vi "interfaz-grafica.vi"() -> ()   [LabVIEW 2024]
uses:
  TG JD - running/TG Juan Diego/Documentos de Labview/160620 Optotune Lens Driver 4 Labview package/Hello Optotune Lens (30.06.2015)/Calibration.ctl
  <vilib>/Instr/_visa.llb/VISA Configure Serial Port (Instr).vi
  <vilib>/Utility/file.llb/Write Delimited Spreadsheet (string).vi
  <vilib>/Utility/file.llb/Read Delimited Spreadsheet (string).vi
  <vilib>/vision/NI_Vision_Development_Module.lvlib
panel:
  out "Path Video":path
  out "Path Potencia Optica D":path
  out "Path Potencia Optica I":path
  in  "stop":bool
  out "Array 2":dbl[](array[numeric])
  out "Array":dbl[](array[numeric])
  out "Path DATOS":path
  in  "stop 2":bool
  out "Path":path=path "C:/Users/willi/GITHUB/TG/OBJ 2 - RECOLECCION DE DATOS/registro-usuarios.csv"
  out "error out":errorcluster
  in  "Tab Control":enum32{"Experimento", "Configuración"}(tab)
  in  "ADQUIRIR":bool
  in  "DETENER":bool
  out "DPT  IZQ":dbl
  out "DPT  DER":dbl
  out "Potencia  Ojo Derecho":dbl[](graph)
  out "ROI (Ojo)":T1(plugin-control)
  out "Path ADQUISICION":path
  out "Usuario seleccionado":string caption="USUARIO"
  in  "Potencia inicial lente derecho":dbl(slide) scale=-3.0..3.0
  in  "Potencia inicial lente izquierdo":dbl(slide) scale=-3.0..3.0
  out "Full Image":T1(plugin-control)
  in  "VISA resource name 3":refnum<visa-resource-name>
  in  "Tab Control 2":T2(tab)
  in  "Usuario":string(combo)
  in  "registrarButtom":bool
  in  "Cluster":T3 {"Fecha de nacimiento" format="%<%x>T"}
  out "Nuevo Usuario":i32
  out "USUARIO":string
  in  "VISA resource name 4":refnum<visa-resource-name>
  out "error out 4":errorcluster
  out "error out 3":errorcluster
  in  "stop 4":bool
  in  "error in (no error) 3":errorcluster
  in  "error in (no error) 4":errorcluster
  in  "stop 3":bool
  out "VISA resource name out 2":string
  out "Command to Port":string
  out "Data":string
  out "OK":bool
  out "Calibration 2":T4 {"Max Current A" format="%#_g mA"; "Max Current B" format="%#_g mA"; "UCL A" format="%#_g mA"; "LCL A" format="%#_g mA"; "UCL B" format="%#_g mA"; "LCL B" format="%#_g mA"}
  out "VISA resource name out":string
  out "ID":u16
  in  "Calibration":T4={"Max Current A"=293.0, "Max Current B"=293.0, "UCL A"=300.0, "UCL B"=300.0, "LCL A"=0.0, "LCL B"=0.0} {"Max Current A" format="%#_g mA"; "Max Current B" format="%#_g mA"; "UCL A" format="%#_g mA"; "LCL A" format="%#_g mA"; "UCL B" format="%#_g mA"; "LCL B" format="%#_g mA"}
  # "Seleccione la Region de Interes (ROI. el ojo)"
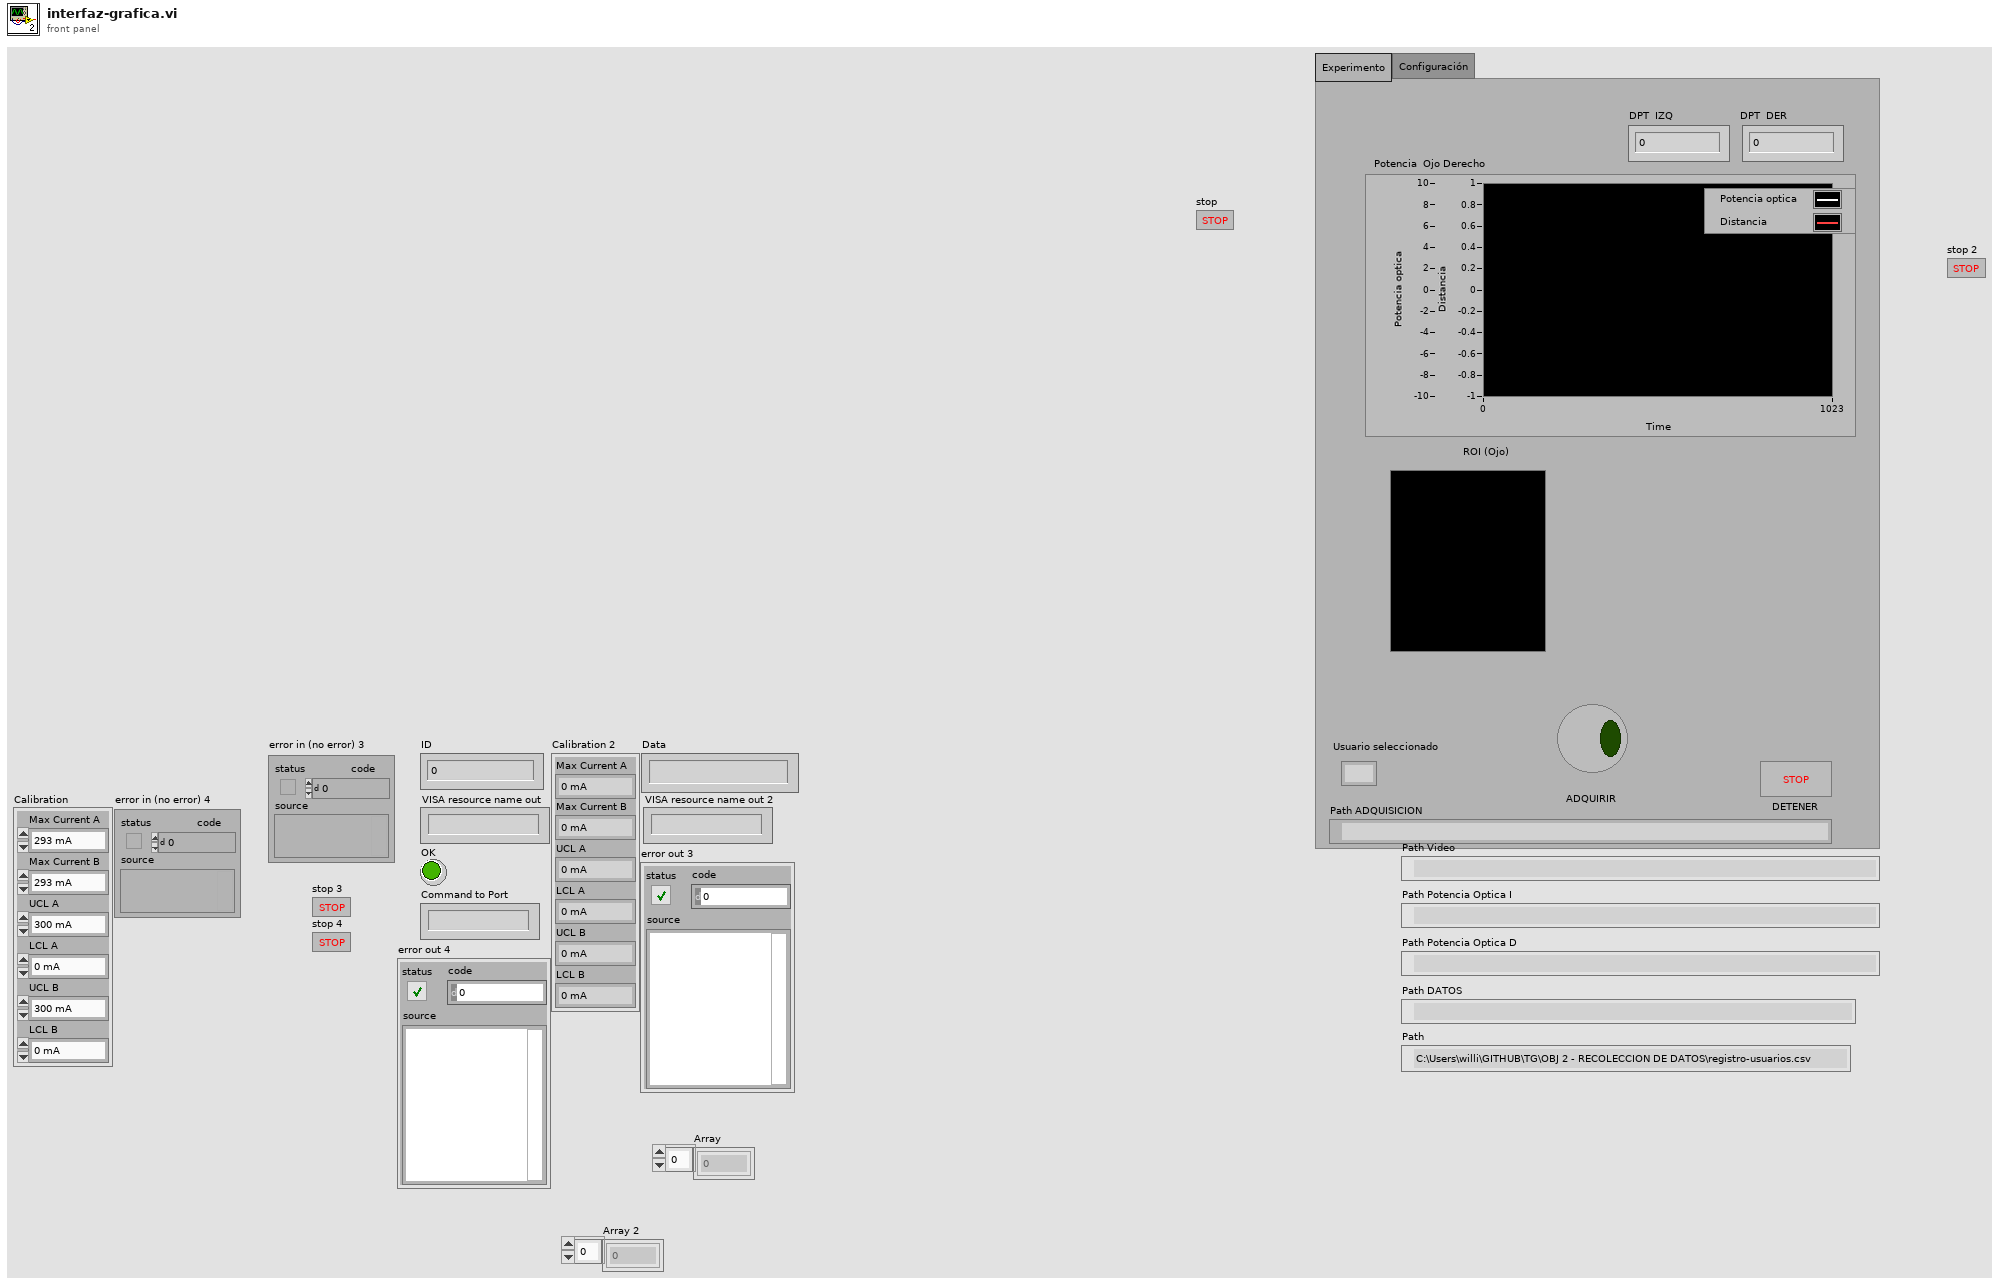
[diagram p1: front panel]
types:
  T1 = typedef "IMAQ Image.ctl" = refnum<image>
  T2 = enum32{"Seleccionar Usuario", "Registrar Nuevo Usuario"}
  T3 = cluster{"Fecha de nacimiento":timestamp, "Genero":enum16{"Mujer", "Hombre"}, "Error Refractivo":enum16{"No sabe", "Miopia", "Hipermetropia", "No tiene"}}
  T4 = typedef "Calibration.ctl" = cluster{"Max Current A":dbl, "Max Current B":dbl, "UCL A":dbl, "UCL B":dbl, "LCL A":dbl, "LCL B":dbl}
  T5 = typedef "Image Type" = u32
  T6 = cluster{"Numero \nUsuario":i32, "Fecha de nacimiento":timestamp, "Genero":enum16{"Mujer", "Hombre"}, "Error Refractivo":enum16{"No sabe", "Miopia", "Hipermetropia", "No tiene"}}
  T7 = enum16{"No sabe", "Miopia", "Hipermetropia", "No tiene"}
  T8 = cluster{"Global Rectangle":i32[], "Contours":cluster{"Contour Type":u32, "ROI Type":u32, "Points":i32[]}[]}
  T9 = typedef "IMAQ AVI2 Refnum.ctl" = refnum<k20>
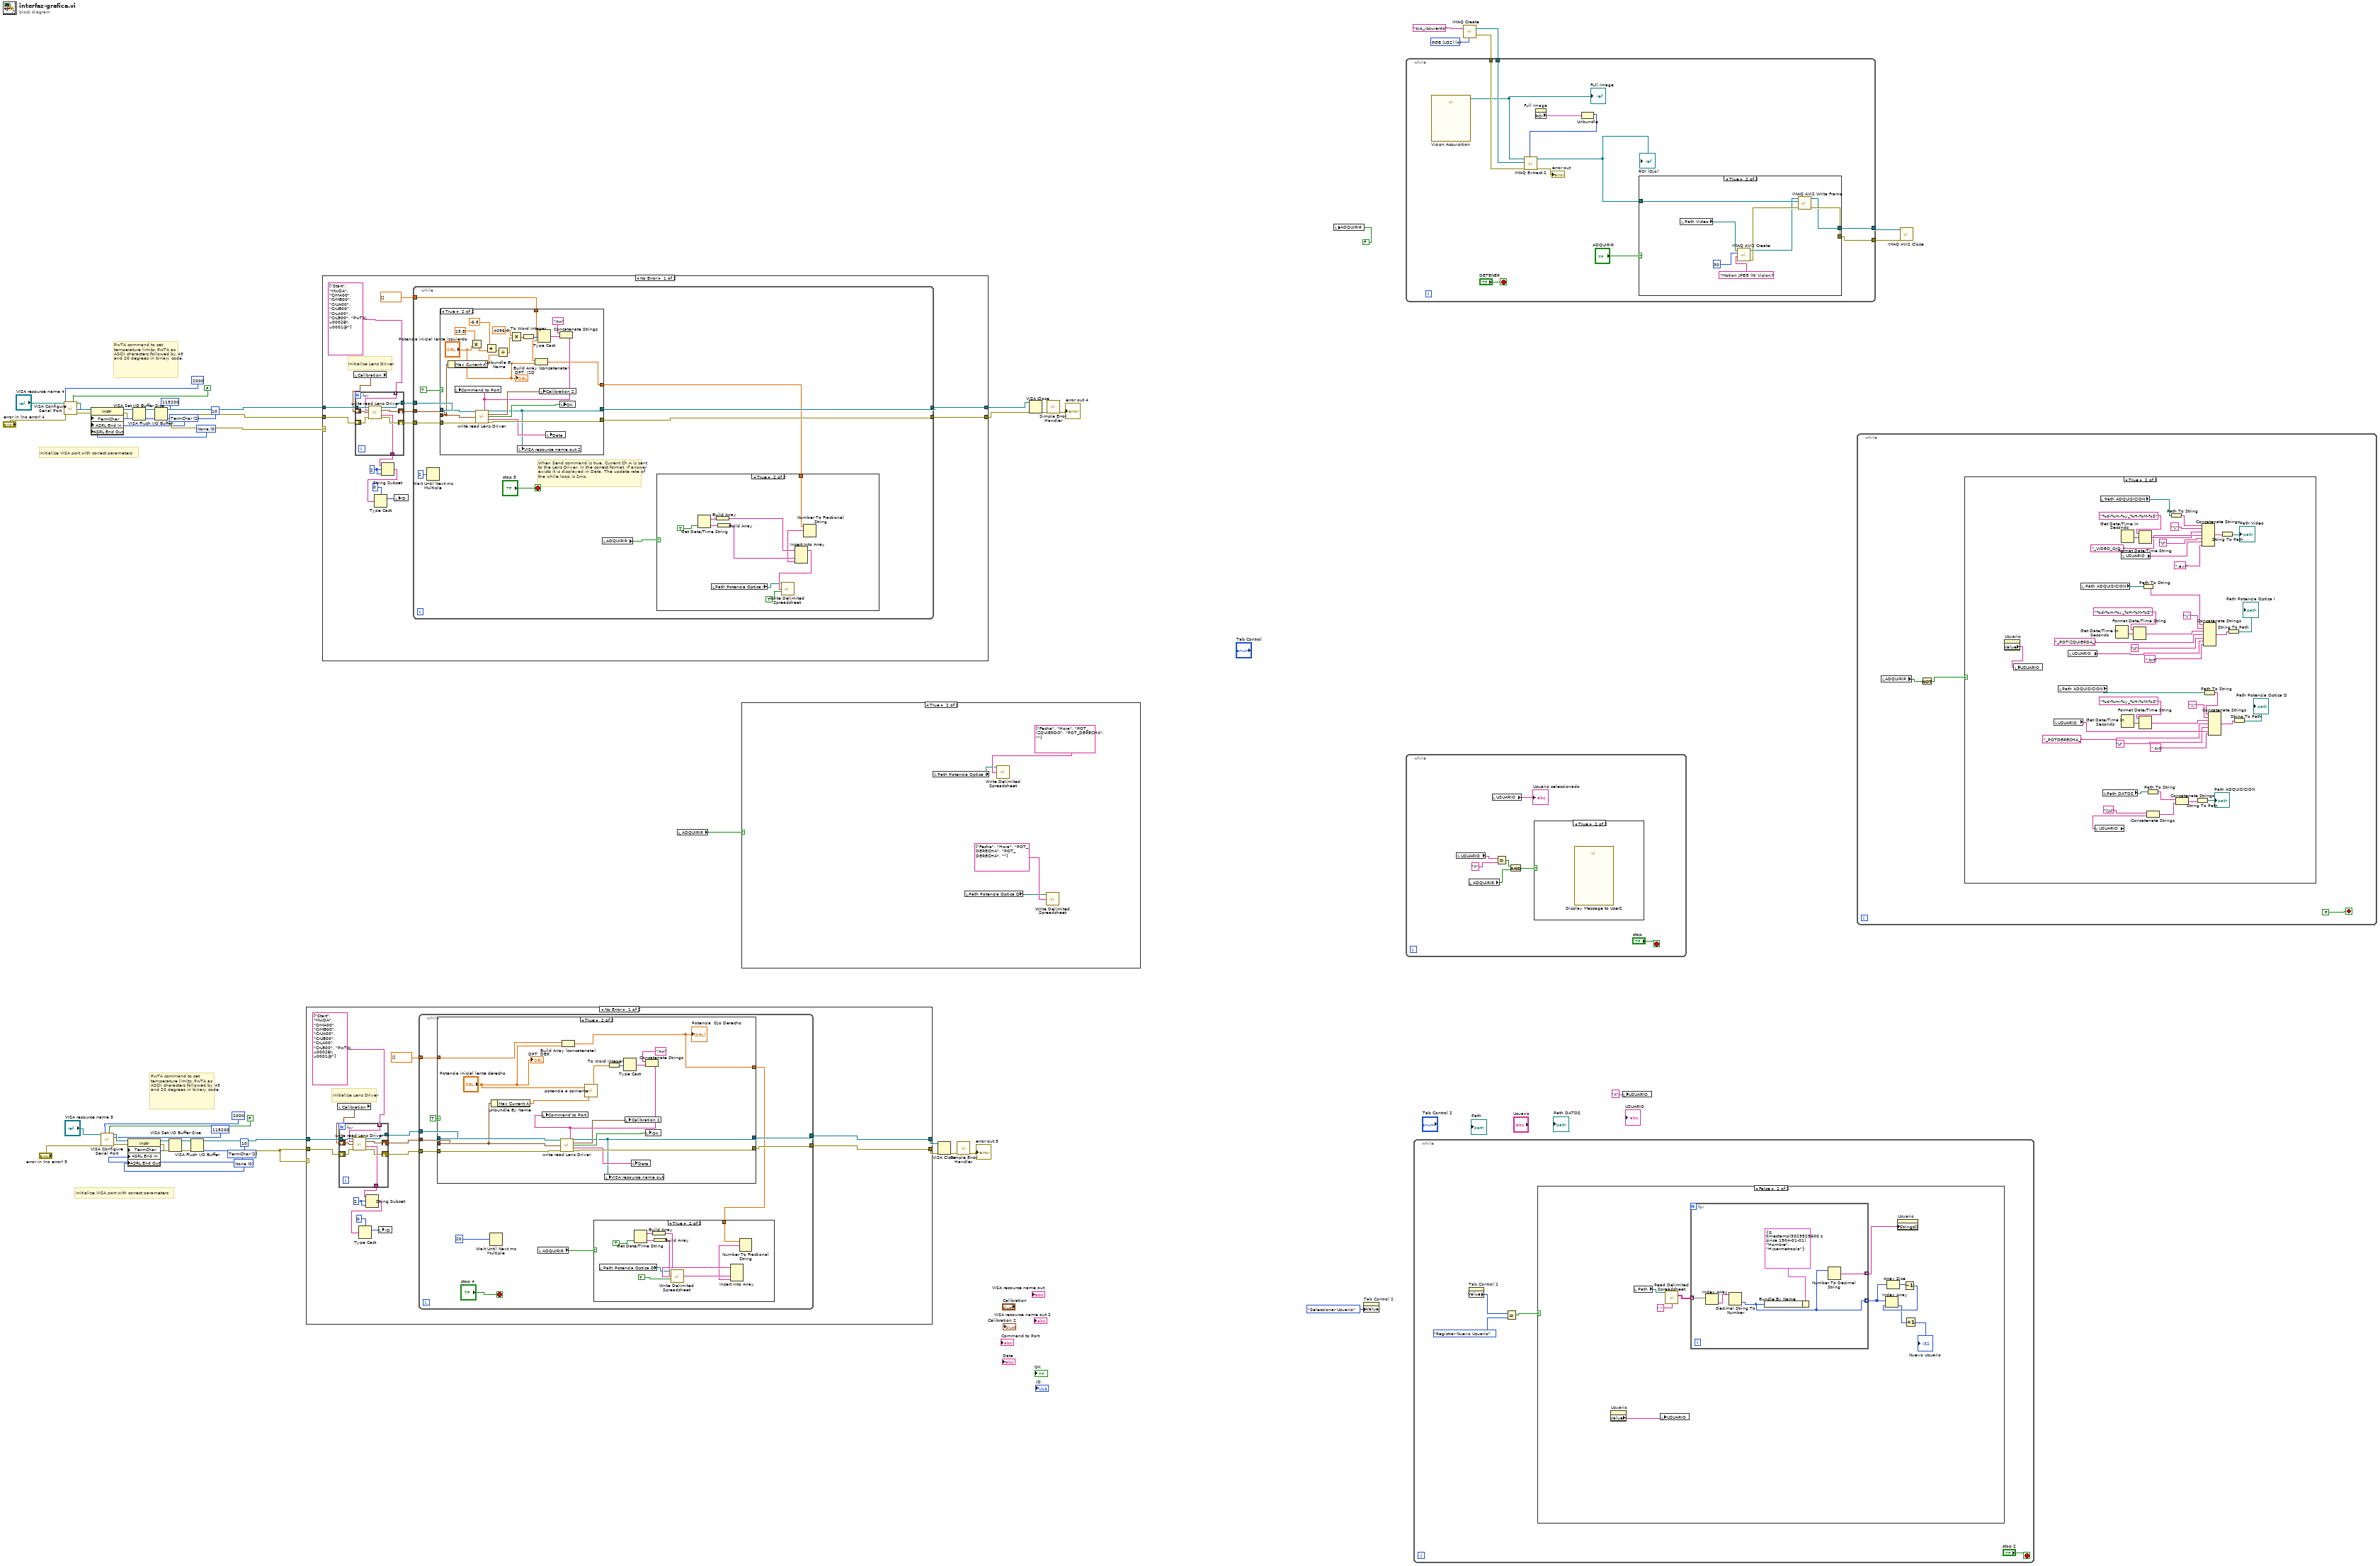
[diagram p0: block diagram]
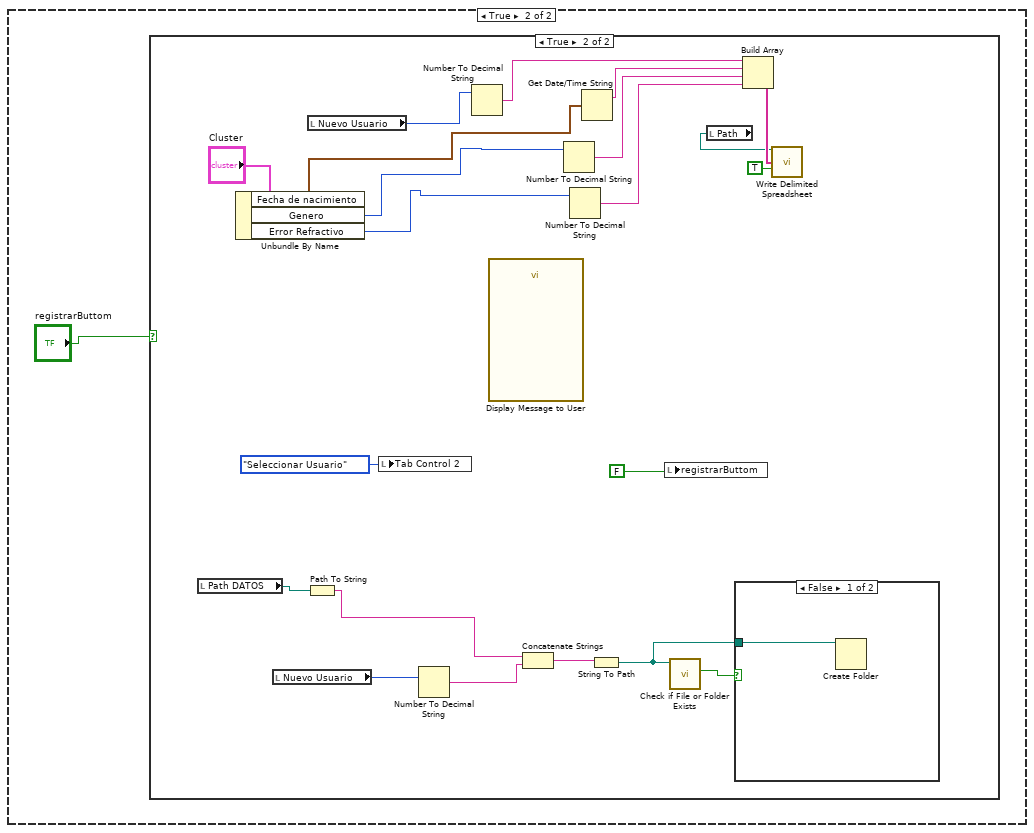
[diagram p5: hidden frame]
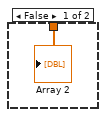
[diagram p9: hidden frame]
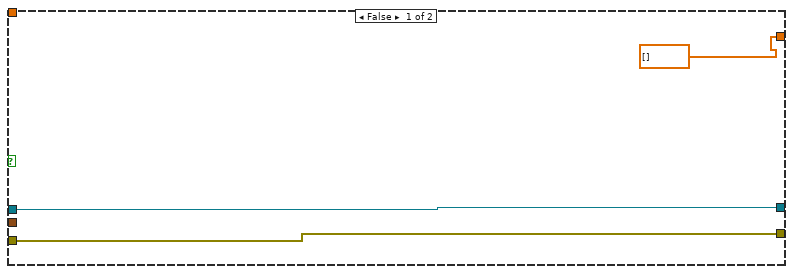
[diagram p10: hidden frame]
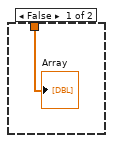
[diagram p12: hidden frame]
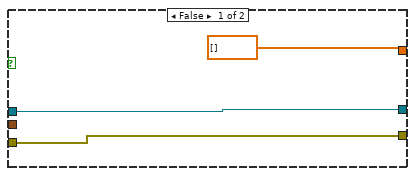
[diagram p13: hidden frame]
diagram:
  w11 = T5 4 items=["Grayscale (U8)", "Grayscale (I16)", "Grayscale (SGL)", "Complex (CSG)", "RGB (U32)", "HSL (U32)", "RGB (U64)", "Grayscale (U16)"] ("Image Type")
  w32 = u16 0 items=["None", "Last Bit", "TermChar", "Break"] ("Serial Settings:End Mode for Writes")
  w31 = u16 2 items=["None", "Last Bit", "TermChar"] ("Serial Settings:End Mode for Reads")
  w44 = u16 0 items=["None", "Last Bit", "TermChar", "Break"] ("Serial Settings:End Mode for Writes")
  w43 = u16 2 items=["None", "Last Bit", "TermChar"] ("Serial Settings:End Mode for Reads")
  # "PwTA command to set temperature limits: PwTA as ASCII characters followed by 45 and 20 degrees in binary code."
  # "Initialize VISA port with correct parameters"
  # "PwTA command to set temperature limits: PwTA as ASCII characters followed by 45 and 20 degrees in binary code."
  # "Initialize VISA port with correct parameters"
  n1 = call-poly "VISA Configure Serial Port"("VISA resource name"="VISA resource name 4", "timeout (10sec)"=u32 2000, "Enable Termination\nChar (T)"=FALSE ("Enable Termination\nChar (T)"), "baud rate (9600)"=u32 115200, "error in (no error)"="error in (no error) 4") -> ("VISA resource name out"=w39:refnum<visa-resource-name>, "error out"=w41:errorcluster)  [unwired: 9 in]
  n2 = property class="Instr"(reference=w39, error in=w41, "TermChar"=u8 10 ("Message Based Settings:Termination Character"), "ASRL End In"=w43, "ASRL End Out"=w44) -> (reference out=w40:refnum<visa-resource-name>, error out=w42:errorcluster)
  n3 = call-poly "VISA Configure Serial Port"("VISA resource name"="VISA resource name 3", "timeout (10sec)"=u32 2000, "Enable Termination\nChar (T)"=FALSE ("Enable Termination\nChar (T)"), "baud rate (9600)"=u32 115200, "error in (no error)"="error in (no error) 3") -> ("VISA resource name out"=w27:refnum<visa-resource-name>, "error out"=w29:errorcluster)  [unwired: 9 in]
  n4 = property class="Instr"(reference=w27, error in=w29, "TermChar"=u8 10 ("Message Based Settings:Termination Character"), "ASRL End In"=w31, "ASRL End Out"=w32) -> (reference out=w28:refnum<visa-resource-name>, error out=w30:errorcluster)
  n5 = VISA Set I/O Buffer Size(VISA resource name=w40, error in (no error)=w42) -> (VISA resource name out=w46:refnum<visa-resource-name>, error out=w47:errorcluster)  [unwired: 2 in]
  n6 = VISA Flush I/O Buffer(VISA resource name=w46, error in (no error)=w47) -> (VISA resource name out=w49:refnum<visa-resource-name>, error out=w48:errorcluster)  [unwired: 1 in]
  n7 = VISA Set I/O Buffer Size(VISA resource name=w28, error in (no error)=w30) -> (VISA resource name out=w34:refnum<visa-resource-name>, error out=w35:errorcluster)  [unwired: 2 in]
  n8 = VISA Flush I/O Buffer(VISA resource name=w34, error in (no error)=w35) -> (VISA resource name out=w22:refnum<visa-resource-name>, error out=w21:errorcluster)  [unwired: 1 in]
  n9 = case shown="No Error" w21 {
    tunnel: w21 -> [w65 w116]
    tunnel: w22 -> [w64 w117]
    tunnel: [w63 w116] -> w17
    tunnel: [w62 w117] -> w18
    frame No Error {
      w61 = 2 ("length (rest)")
      # "Initialize Lens Driver"
      n10 = local read "Calibration"() -> (w53:T4)
      n11 = for {
        tunnel: w64 -> [w114]
        tunnel: [w111] -> w56
        tunnel: string[] ["Start", "MwDA", "CrMA00", "CrMB00", "CrUA00", "CrUB00", "CrLA00", "CrLB00", "PwTA\u0002Ð\u0001@"] -> [w109] mode=indexing
        tunnel: [w108] -> w55
        shift-right: [w112] -> w57
        shift-left: w53 -> [w113]
        shift-right: [w110] -> w58
        shift-left: w65 -> [w115]
        n12 = call "write read Lens Driver.vi"("VISA resource name"=w114, "command"=w109, "Calibration"=w113, "error in (no error)"=w115) -> ("VISA resource name out"=w111:refnum<visa-resource-name>, "Calibration 2"=w112:T4, "Data"=w108:string, "error out"=w110:errorcluster)  [unwired: 4 in, 4 out]
      }
      n13 = String Subset(string=w55, offset (0)=w61, length (rest)=w61) -> (substring=w59:string)
      n14 = Type Cast(type=u16 0 ("length (rest)"), x=w59) -> (*(type *) &x=w54:u16)
      n15 = local write "ID"(w54) -> ()
      n16 = while {
        tunnel: [w70] -> w63
        tunnel: [w71] -> w62
        tunnel: w58 -> [w76]
        tunnel: w57 -> [w75]
        tunnel: w56 -> [w74]
        tunnel: dbl[] [] -> [w68]
        stop <- "stop 4" stop-if-true
        n17 = case shown="True" TRUE ("Send command") {
          tunnel: [w90 w107] -> w70
          tunnel: w76 -> [w90 w106]
          tunnel: w75 -> [_ w97]
          tunnel: w74 -> [w89 w105]
          tunnel: [w89 w98] -> w71
          tunnel: w68 -> [_ w92]
          tunnel: [dbl[] [] w91] -> w67
          frame False {
          }
          frame True {
            n18 = Unbundle By Name(w97) -> ("Max Current A"=w96:dbl)
            n19 = Build Array (concatenate)(w92, "Potencia inicial lente derecho") -> (w91:dbl[])
            "Potencia  Ojo Derecho" <- w91
            n20 = call "potencia a corriente.vi"("Max current A"=w96, "Potencia"="Potencia inicial lente derecho") -> ("Corriente"=w95:dbl)
            n21 = To Word Integer(number=w95) -> (16bit integer=w104:i16)
            n22 = Type Cast(x=w104) -> (*(type *) &x=w103:string)  [unwired: 1 in]
            n23 = Concatenate Strings("Aw", w103) -> (w100:string)
            n24 = local write "Command to Port"(w100) -> ()
            n25 = call "write read Lens Driver.vi"("VISA resource name"=w105, "command"=w100, "Calibration"=w97, "error in (no error)"=w106) -> ("VISA resource name out"=w98:refnum<visa-resource-name>, "Calibration 2"=w102:T4, "OK"=w101:bool, "Data"=w99:string, "error out"=w107:errorcluster)  [unwired: 4 in, 3 out]
            n26 = local write "VISA resource name out"(w98) -> ()
            n27 = local write "Calibration 2"(w102) -> ()
            n28 = local write "Data"(w99) -> ()
            n29 = local write "OK"(w101) -> ()
            "DPT  DER" <- "Potencia inicial lente derecho"
          }
        }
        n30 = Wait Until Next ms Multiple(millisecond multiple=u32 20) -> ()  [unwired: 1 out]
        n31 = local read "ADQUIRIR"() -> (w66:bool)
        n32 = case shown="True" w66 {
          tunnel: w67 -> [w77 w79]
          frame False {
            "Array 2" <- w77
          }
          frame True {
            n33 = local read "Path Potencia Optica D"() -> (w78:path)
            n34 = Get Date/Time String(want seconds? (F)=TRUE) -> (date string=w87:string, time string=w86:string)  [unwired: 2 in]
            n35 = Build Array(w87) -> (w85:string[])
            n36 = Build Array(w86) -> (w84:string[])
            n37 = Number To Fractional String(number=w79) -> (F-format string=w80:string[])  [unwired: 3 in]
            n38 = Insert Into Array(array=w85, new element #1=w84, new element #2=w80) -> (w83:string[])  [unwired: 1 in]
            n39 = call-poly <vilib>:"Write Delimited Spreadsheet.vi"("file path (dialog if empty)"=w78, "1D data"=w83, "append to file? (new file:F)"=TRUE) -> ()  [unwired: 11 in, 2 out]
          }
        }
      }
    }
    frame Error {
    }
  }
  n40 = case shown="No Error" w48 {
    tunnel: w48 -> [w132 w189]
    tunnel: w49 -> [w131 w190]
    tunnel: [w130 w189] -> w14
    tunnel: [w129 w190] -> w13
    frame No Error {
      w128 = 2 ("length (rest)")
      # "Initialize Lens Driver"
      n41 = local read "Calibration"() -> (w120:T4)
      n42 = for {
        tunnel: w131 -> [w187]
        tunnel: [w184] -> w123
        tunnel: string[] ["Start", "MwDA", "CrMA00", "CrMB00", "CrUA00", "CrUB00", "CrLA00", "CrLB00", "PwTA\u0002Ð\u0001@"] -> [w182] mode=indexing
        tunnel: [w181] -> w122
        shift-right: [w185] -> w124
        shift-left: w120 -> [w186]
        shift-right: [w183] -> w125
        shift-left: w132 -> [w188]
        n43 = call "write read Lens Driver.vi"("VISA resource name"=w187, "command"=w182, "Calibration"=w186, "error in (no error)"=w188) -> ("VISA resource name out"=w184:refnum<visa-resource-name>, "Calibration 2"=w185:T4, "Data"=w181:string, "error out"=w183:errorcluster)  [unwired: 4 in, 4 out]
      }
      n44 = String Subset(string=w122, offset (0)=w128, length (rest)=w128) -> (substring=w126:string)
      n45 = Type Cast(type=u16 0 ("length (rest)"), x=w126) -> (*(type *) &x=w121:u16)
      n46 = local write "ID"(w121) -> ()
      n47 = while {
        tunnel: [w137] -> w130
        tunnel: [w138] -> w129
        tunnel: w125 -> [w143]
        tunnel: w124 -> [w142]
        tunnel: w123 -> [w141]
        tunnel: dbl[] [] -> [w134]
        stop <- "stop 3" stop-if-true
        # "When Send command is true, Current Ch A is sent to the Lens Driver, in the correct format. If answer exists it is displayed in Data. The update rate of the while loop is 2ms."
        n48 = Wait Until Next ms Multiple(millisecond multiple=u32 2) -> ()  [unwired: 1 out]
        n49 = case shown="True" TRUE ("Send command") {
          tunnel: [w157 w180] -> w137
          tunnel: w143 -> [w157 w179]
          tunnel: w142 -> [_ w167]
          tunnel: w141 -> [w156 w178]
          tunnel: [w156 w168] -> w138
          tunnel: [dbl[] [] w158] -> w135
          tunnel: w134 -> [_ w160]
          frame False {
          }
          frame True {
            n50 = Unbundle By Name(w167) -> ("Max Current A"=w166:dbl)
            n51 = Multiply(x=15.8, y="Potencia inicial lente izquierdo") -> (x*y=w164:dbl)
            n52 = Add(x=-6.8, y=w164) -> (x+y=w162:dbl)
            n53 = Divide(x=w162, y=w166) -> (x/y=w165:dbl)
            n54 = Multiply(x=4096.0, y=w165) -> (x*y=w176:dbl)
            n55 = To Word Integer(number=w176) -> (16bit integer=w175:i16)
            n56 = Build Array (concatenate)(w160, "Potencia inicial lente izquierdo") -> (w158:dbl[])
            n57 = Type Cast(x=w175) -> (*(type *) &x=w174:string)  [unwired: 1 in]
            n58 = Concatenate Strings("Aw", w174) -> (w170:string)
            n59 = local write "Command to Port"(w170) -> ()
            n60 = call "write read Lens Driver.vi"("VISA resource name"=w178, "command"=w170, "Calibration"=w167, "error in (no error)"=w179) -> ("VISA resource name out"=w168:refnum<visa-resource-name>, "Calibration 2"=w172:T4, "OK"=w171:bool, "Data"=w169:string, "error out"=w180:errorcluster)  [unwired: 4 in, 3 out]
            n61 = local write "VISA resource name out 2"(w168) -> ()
            n62 = local write "Calibration 2"(w172) -> ()
            n63 = local write "Data"(w169) -> ()
            n64 = local write "OK"(w171) -> ()
            "DPT  IZQ" <- "Potencia inicial lente izquierdo"
          }
        }
        n65 = local read "ADQUIRIR"() -> (w133:bool)
        n66 = case shown="True" w133 {
          tunnel: w135 -> [w144 w146]
          frame False {
            "Array" <- w144
          }
          frame True {
            n67 = Get Date/Time String(want seconds? (F)=TRUE) -> (date string=w154:string, time string=w153:string)  [unwired: 2 in]
            n68 = local read "Path Potencia Optica I"() -> (w145:path)
            n69 = Build Array(w154) -> (w152:string[])
            n70 = Build Array(w153) -> (w151:string[])
            n71 = Number To Fractional String(number=w146) -> (F-format string=w147:string[])  [unwired: 3 in]
            n72 = Insert Into Array(array=w152, new element #1=w151, new element #2=w147) -> (w150:string[])  [unwired: 1 in]
            n73 = call-poly <vilib>:"Write Delimited Spreadsheet.vi"("file path (dialog if empty)"=w145, "1D data"=w150, "append to file? (new file:F)"=TRUE) -> ()  [unwired: 11 in, 2 out]
          }
        }
      }
    }
    frame Error {
    }
  }
  n74 = local read "ADQUIRIR"() -> (w2:bool)
  n75 = case shown="True" w2 {
    frame False {
    }
    frame True {
      n76 = local read "Path Potencia Optica I"() -> (w192:path)
      n77 = local read "Path Potencia Optica D"() -> (w191:path)
      n78 = call-poly <vilib>:"Write Delimited Spreadsheet.vi"("file path (dialog if empty)"=w192, "1D data"=string[] ["Fecha", "Hora", "POT_IZQUIERDO", "POT_DERECHA", ""]) -> ()  [unwired: 12 in, 2 out]
      n79 = call-poly <vilib>:"Write Delimited Spreadsheet.vi"("file path (dialog if empty)"=w191, "1D data"=string[] ["Fecha", "Hora", "POT_DERECHA", "POT_DERECHA", ""]) -> ()  [unwired: 12 in, 2 out]
    }
  }
  n80 = VISA Close(VISA resource name=w18, error in (no error)=w17) -> (error out=w20:errorcluster)
  n81 = call <vilib>:"Simple Error Handler.vi"("error in (no error)"=w20) -> ("error out"=→"error out 3":errorcluster)  [unwired: 4 in, 4 out]
  n82 = VISA Close(VISA resource name=w13, error in (no error)=w14) -> (error out=w16:errorcluster)
  n83 = call <vilib>:"Simple Error Handler.vi"("error in (no error)"=w16) -> ("error out"=→"error out 4":errorcluster)  [unwired: 4 in, 4 out]
  n84 = local write "ADQUIRIR"(FALSE ("ADQUIRIR")) -> ()
  n85 = property on="Tab Control 2" class="TabCtl (strict)"("Value"=T2."Seleccionar Usuario" ("Tab Control 2")) -> ()  [unwired: 2 in, 2 out]
  n86 = while {
    stop <- "stop" stop-if-true
    n87 = local read "USUARIO"() -> (w196:string)
    n88 = local read "ADQUIRIR"() -> (w198:bool)
    n89 = local read "USUARIO"() -> (→"Usuario seleccionado":string)
    n90 = Equal?(x=w196, y="X") -> (x = y?=w197:bool)
    n91 = And(x=w197, y=w198) -> (x .and. y?=w199:bool)
    n92 = case shown="True" w199 {
      frame False {
      }
      frame True {
        n93 = call "Display Message to User2"() -> ()  [unwired: 10 in, 2 out]
      }
    }
  }
  n94 = while {
    stop <- "stop 2" stop-if-true
    n95 = property on="Tab Control 2" class="TabCtl (strict)"() -> ("Value"=w204:T2)  [unwired: 2 in, 2 out]
    n96 = Equal?(x=w204, y=T2."Registrar Nuevo Usuario") -> (x = y?=w205:bool)
    n97 = case shown="False" w205 {
      frame False {
        n98 = property on="Usuario" class="CmbBox"() -> ("Value"=w206:string)  [unwired: 2 in, 2 out]
        n99 = local read "Path"() -> (w214:path)
        n100 = local write "USUARIO"(w206) -> ()
        n101 = call-poly <vilib>:"Read Delimited Spreadsheet.vi"("file path (dialog if empty)"=w214, "delimiter (\\t)"="," ("delimiter (\\t)")) -> ("all rows"=w213:string[][])  [unwired: 8 in, 5 out]
        n102 = for {
          tunnel: w213 -> [w220] mode=indexing
          tunnel: [w217] -> w212 mode=indexing
          tunnel: [w216] -> w207 mode=indexing
          n103 = Index Array(array=w220) -> (element=w218:string)  [unwired: 1 in]
          n104 = Decimal String To Number(string=w218) -> (number=w217:i32)  [unwired: 2 in, 1 out]
          n105 = Bundle By Name(cluster=T6 {"Numero \nUsuario"=0, "Fecha de nacimiento"=timestamp(3029529600 s since 1904-01-01), "Genero"=enum."Hombre", "Error Refractivo"=enum."Hipermetropia"} ("Cluster"), "Numero \nUsuario"=w217) -> ()  [unwired: 1 out]
          n106 = Number To Decimal String(number=w217) -> (decimal integer string=w216:string)  [unwired: 1 in]
        }
        n107 = Array Size(array=w212) -> (size(s)=w211:i32)
        n108 = property on="Usuario" class="CmbBox"("Strings[]"=w207) -> ()  [unwired: 2 in, 2 out]
        n109 = Decrement(x=w211) -> (x-1=w210:i32)
        n110 = Index Array(array=w212, index=w210) -> (element=w209:i32)
        n111 = Increment(x=w209) -> (x+1=→"Nuevo Usuario":i32)
      }
      frame True {
        n112 = case shown="True" "registrarButtom" {
          frame False {
          }
          frame True {
            n113 = local read "Path DATOS"() -> (w223:path)
            n114 = Unbundle By Name("Cluster") -> ("Fecha de nacimiento"=w232:timestamp, "Genero"=w231:enum16{"Mujer", "Hombre"}, "Error Refractivo"=w230:T7)
            n115 = local read "Nuevo Usuario"() -> (w228:i32)
            n116 = Path To String(path=w223) -> (string=w222:string)
            n117 = local read "Nuevo Usuario"() -> (w229:i32)
            n118 = local write "Tab Control 2"(T2."Seleccionar Usuario" ("Tab Control 2")) -> ()
            n119 = Number To Decimal String(number=w228) -> (decimal integer string=w227:string)  [unwired: 1 in]
            n120 = Number To Decimal String(number=w229) -> (decimal integer string=w237:string)  [unwired: 1 in]
            n121 = call "Display Message to User"() -> ()  [unwired: 10 in, 2 out]
            n122 = Concatenate Strings(w222, w227) -> (w226:string)
            n123 = Number To Decimal String(number=w231) -> (decimal integer string=w235:string)  [unwired: 1 in]
            n124 = Number To Decimal String(number=w230) -> (decimal integer string=w234:string)  [unwired: 1 in]
            n125 = Get Date/Time String(seconds (now)=w232) -> (date string=w236:string)  [unwired: 2 in, 1 out]
            n126 = String To Path(string=w226) -> (path=w225:path)
            n127 = local write "registrarButtom"(FALSE ("registrarButtom")) -> ()
            n128 = call <vilib>:"Check if File or Folder Exists.vi"("path"=w225) -> ("file or folder exists?"=w224:bool)  [unwired: 8 in, 2 out]
            n129 = local read "Path"() -> (w241:path)
            n130 = case shown="False" w224 {
              tunnel: w225 -> [w243 _]
              frame False {
                n131 = Create Folder(path (use dialog)=w243) -> ()  [unwired: 2 in, 3 out]
              }
              frame True {
              }
            }
            n132 = Build Array(w237, w236, w235, w234) -> (w242:string[])
            n133 = call-poly <vilib>:"Write Delimited Spreadsheet.vi"("file path (dialog if empty)"=w241, "1D data"=w242, "append to file? (new file:F)"=TRUE) -> ()  [unwired: 11 in, 2 out]
          }
        }
      }
    }
  }
  n134 = call "IMAQ Create"("Image Name"="ojo_izquierdo", "Image Type"=w11) -> ("New Image"=w9:T1, "error out"=w10:errorcluster)  [unwired: 3 in]
  n135 = while {
    tunnel: w10 -> [w253]
    tunnel: w9 -> [w252]
    tunnel: [w245] -> w8
    tunnel: [w244] -> w7
    stop <- "DETENER" stop-if-true
    n136 = call "Vision Acquisition"() -> ("Image Out"=w248:T1)  [unwired: 25 in, 2 out]
    "Full Image" <- w248
    n137 = property on="Full Image" class="ImageControl"() -> ("ROI"=w251:T8)  [unwired: 2 in, 2 out]
    n138 = Unbundle "Unbundle"(w251) -> ("Global Rectangle"=w250:i32[])  [unwired: 1 out]
    n139 = call "IMAQ Extract 2"("Optional Rectangle"=w250, "error in (no error)"=w253, "Image Dst"=w252, "Image Src"=w248) -> ("error out"=→"error out":errorcluster, "Image Dst Out"=w246:T1)  [unwired: 6 in]
    "ROI (Ojo)" <- w246
    n140 = case shown="True" "ADQUIRIR" {
      tunnel: [_ w262] -> w245
      tunnel: [_ w261] -> w244
      tunnel: w246 -> [_ w260]
      frame False {
      }
      frame True {
        n141 = local read "Path Video"() -> (w255:path)
        n142 = call "IMAQ AVI2 Create"("Codec"="Motion JPEG (NI Vision)", "Frames Per Second"=u32 30, "AVI Path"=w255) -> ("error out"=w257:errorcluster, "AVI Refnum"=w256:T9)  [unwired: 7 in]
        n143 = call "IMAQ AVI2 Write Frame"("error in (no error)"=w257, "Image"=w260, "AVI Refnum"=w256) -> ("error out"=w262:errorcluster, "AVI Refnum (duplicate)"=w261:T9)  [unwired: 6 in, 1 out]
      }
    }
  }
  n144 = local write "USUARIO"("X" ("USUARIO")) -> ()
  n145 = while {
    stop <- FALSE ("stop 5") stop-if-true
    n146 = local read "ADQUIRIR"() -> (w264:bool)
    n147 = Not(x=w264) -> (.not. x?=w263:bool)
    n148 = case shown="True" w263 {
      frame False {
      }
      frame True {
        n149 = property on="Usuario" class="CmbBox"() -> ("Value"=w266:string)  [unwired: 2 in, 2 out]
        n150 = local write "USUARIO"(w266) -> ()
        n151 = local read "USUARIO"() -> (w302:string)
        n152 = local read "Path ADQUISICION"() -> (w299:path)
        n153 = local read "USUARIO"() -> (w301:string)
        n154 = local read "Path ADQUISICION"() -> (w300:path)
        n155 = local read "USUARIO"() -> (w283:string)
        n156 = local read "Path ADQUISICION"() -> (w309:path)
        n157 = local read "Path DATOS"() -> (w284:path)
        n158 = Get Date/Time In Seconds() -> (seconds since 1Jan1904=w289:timestamp)
        n159 = Get Date/Time In Seconds() -> (seconds since 1Jan1904=w304:timestamp)
        n160 = Get Date/Time In Seconds() -> (seconds since 1Jan1904=w292:timestamp)
        n161 = local read "USUARIO"() -> (w306:string)
        n162 = Format Date/Time String(time format string (%c)="%d-%m-%y_%H-%M-%S", seconds (now)=w289) -> (date/time string=w291:string)  [unwired: 1 in]
        n163 = Format Date/Time String(time format string (%c)="%d-%m-%y_%H-%M-%S", seconds (now)=w304) -> (date/time string=w305:string)  [unwired: 1 in]
        n164 = Format Date/Time String(time format string (%c)="%d-%m-%y_%H-%M-%S", seconds (now)=w292) -> (date/time string=w294:string)  [unwired: 1 in]
        n165 = Path To String(path=w300) -> (string=w295:string)
        n166 = Path To String(path=w284) -> (string=w285:string)
        n167 = Concatenate Strings("\\U" ("string"), w283) -> (w286:string)
        n168 = Path To String(path=w309) -> (string=w303:string)
        n169 = Concatenate Strings(w285, w286) -> (w287:string)
        n170 = String To Path(string=w287) -> (path=→"Path ADQUISICION":path)
        n171 = Concatenate Strings(w303, "\\" ("string"), w305, "_VIDEO_OJO_" ("string"), "U" ("string"), w306, ".avi" ("string")) -> (w307:string)
        n172 = Concatenate Strings(w295, "\\" ("string"), w291, "_POTIZQUIERDA_" ("string"), "U" ("string"), w301, ".txt" ("string")) -> (w290:string)
        n173 = Path To String(path=w299) -> (string=w296:string)
        n174 = Concatenate Strings(w296, "\\" ("string"), w294, "_POTDERECHA_" ("string"), "U" ("string"), w302, ".txt" ("string")) -> (w293:string)
        n175 = String To Path(string=w307) -> (path=→"Path Video":path)
        n176 = String To Path(string=w290) -> (path=→"Path Potencia Optica I":path)
        n177 = String To Path(string=w293) -> (path=→"Path Potencia Optica D":path)
      }
    }
  }
  n178 = call "IMAQ AVI2 Close"("error in (no error)"=w8, "AVI Refnum"=w7) -> ()  [unwired: 9 in, 1 out]
